vi "HandleComands.vi"(0 "Stand in":refnum<class "Stand.lvclass">, 11 "error in (no error)":errorcluster) -> (4 "Stand out":refnum<class "Stand.lvclass">, 6 "String":string, 13 "dt handle cmd":u32, 15 "error out":errorcluster)   [LabVIEW 2019, in "Stand.lvclass"]
uses:
  Stand.lvclass
  C:/Users/ANENKOV_V1/Desktop/src/Device_class/Device.lvclass
  Device_class/Device.lvclass/Device.ctl
  Proccess_class/Proccess.lvclass/Proccess.ctl
  Modbus_class/CMD REG.ctl
  Stand.lvclass/Stand.ctl
  TypeDef/CalibrationData.ctl
  TypeDef/GUI Setting Channel.ctl
  TypeDef/GUI AI Ranges.ctl
  TypeDef/Scale Data.ctl
  SV_Puplisher_class/SV_Publisher.lvclass/SV_Publisher.ctl
  fa7aa4b9-2980-448f-9ea7-f9a96ba04b16.vi
  cf98acac-72aa-4535-b835-e10be751fc5f.vi
  bfc9a858-c3a6-4d13-83b8-6384ea99c5a7.vi
  f74d70ca-5a31-43fe-8564-a719dafc7d08.vi
  9504c8ef-5d3e-4147-8f9a-94e23ec0f1f3.vi
  02f03ceb-97e6-4151-91fa-f86219b8bb60.vi
  cdc27d4a-684e-4578-89c7-fa6de6d60a20.vi
  13e1ba5d-889d-4619-89c4-93477e31edff.vi
  9c9d60f0-6a44-4683-935b-c5188c5c961e.vi
  39aaaa99-a8d8-4d9f-8d69-d9ea65c11964.vi
  1f4e3915-6da8-46a8-831b-0301257cc98b.vi
  46a8ca8a-9e53-4c5b-b4d2-ef9efb1f3638.vi
  12eadd95-888c-421b-8b03-5d7b3a747bbb.vi
  Proccess_class/GetNames.vi
  Proccess_class/GetLogger.vi
  SV_Puplisher_class/Set SV.vi/1ae5d02c-efd0-450a-8aa4-8388e25d05bc.vi
  Device_class/Device.lvclass
  C:/Users/ANENKOV_V1/Desktop/src/Proccess_class/Proccess.lvclass
  Logger_class/WriteEvent.vi
  <vilib>/addons/_JKI.lib/Serialization/JSON/Library/Unflatten From JSON String.vi
  MessageInterface_class/MessageInterface.lvclass
  FPGA_API_class/FPGA API.lvclass
  ConfigInterface_class/ConfigInterface.lvclass
  SV_Puplisher_class/SV_Publisher.lvclass
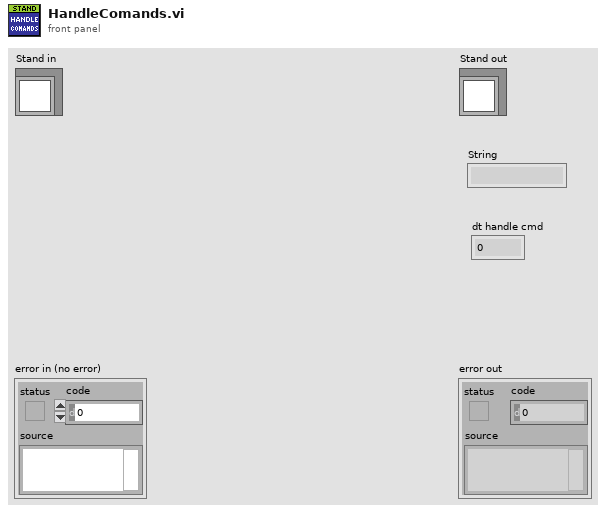
[diagram p1: front panel]
types:
  T1 = typedef "MessageInterface.lvclass/Message.ctl" = cluster{"name":string, "value":string, "receiver host":string, "receiver process":string, "source host":string, "source process":string}
  T2 = typedef "CMD REG.ctl" = cluster{"EXECUTE_SP":bool, "ALARM_PRESS_DOWN_DUT":bool, "ALARM_PRESS_DOWN_CHAMBER":bool, "ALARM_PRESS_DOWN_DUT_CHAMBER":bool, "FILING_DUT":bool, "FILING_CHAMBER":bool, "BLOCK":bool, "PUMP_STATION_OFF":bool, "Leak start":bool, "Leak stop":bool, "Drain":bool}
  T3 = typedef "CalibrationData.ctl" = cluster{"Channels":T4[], "Scales":T6[]}
  T4 = typedef "GUI Setting Channel.ctl" = cluster{"Name":string, "AI Ranges":T5, "ScaleIndex":u32}
  T5 = typedef "GUI AI Ranges.ctl" = cluster{"HI":bool, "HIHI":bool, "LO":bool, "LOLO":bool, "HIHI VAL":dbl, "HI VAL":dbl, "LO VAL":dbl, "LOLO VAL":dbl, "MAX RAW":dbl, "MIN RAW":dbl, "MAX SCALED":dbl, "MIN SCALED":dbl}
  T6 = typedef "Scale Data.ctl" = cluster{"index":i32, "Name":string, "X":dbl[], "Y":dbl[]}
  T7 = typedef "Setting Stand.ctl" = cluster{"Pressure Source":T8, "dt pressure down ms":i32, "dP pressure down MPa":dbl, "Haskel":T9, "Pump":T9, "Accuracy [%]":dbl, "Accuracy max [MPa]":dbl, "Accuracy min [MPa]":dbl, "BackPressurVoltage [V]":dbl}
  T8 = typedef "Pressure Source.ctl" = enum16{"Internal", "Modbus", "UDP"}
  T9 = typedef "Setting Pressure PI.ctl" = cluster{"A [MPa/V]":dbl, "P0 [MPa]":dbl}
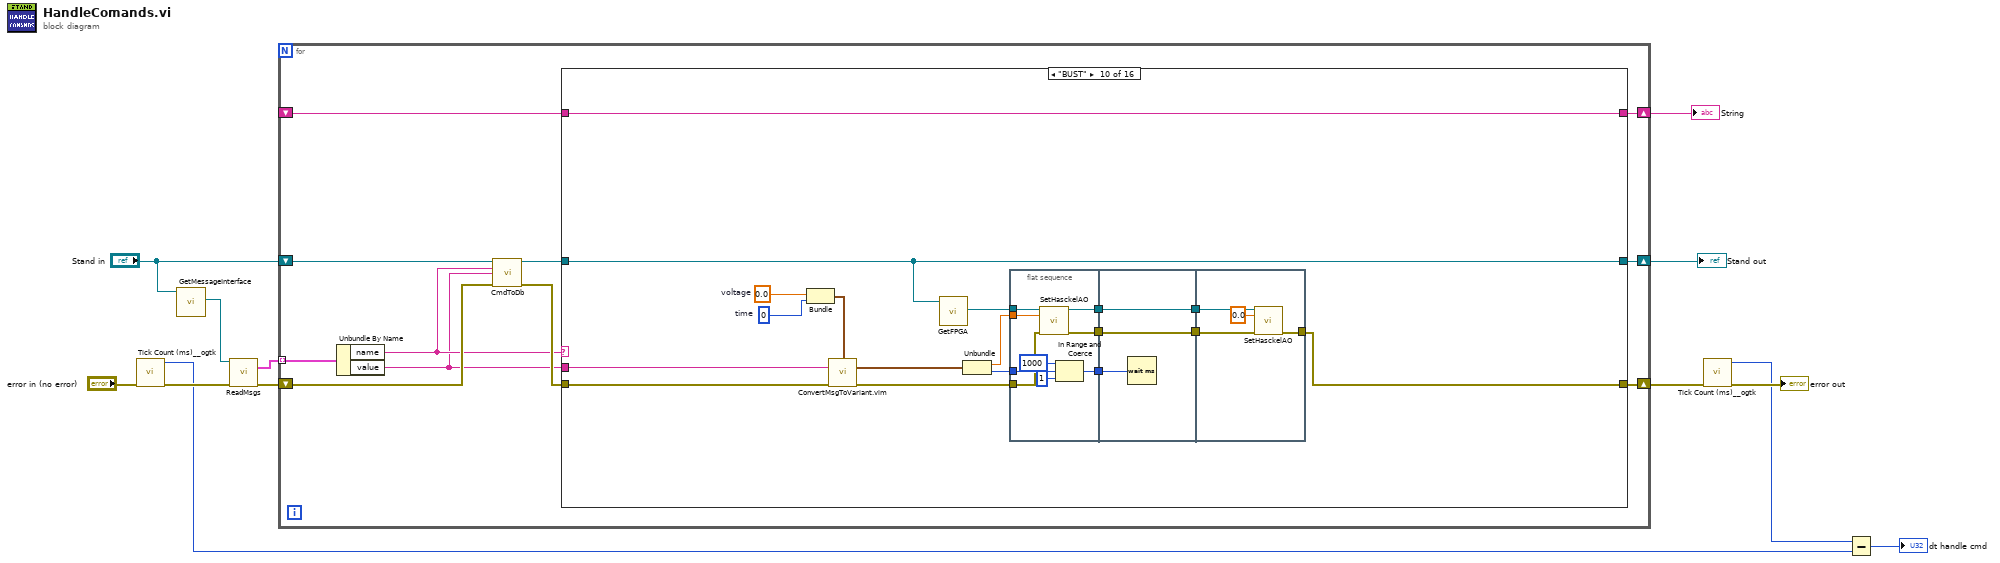
[diagram p0: block diagram]
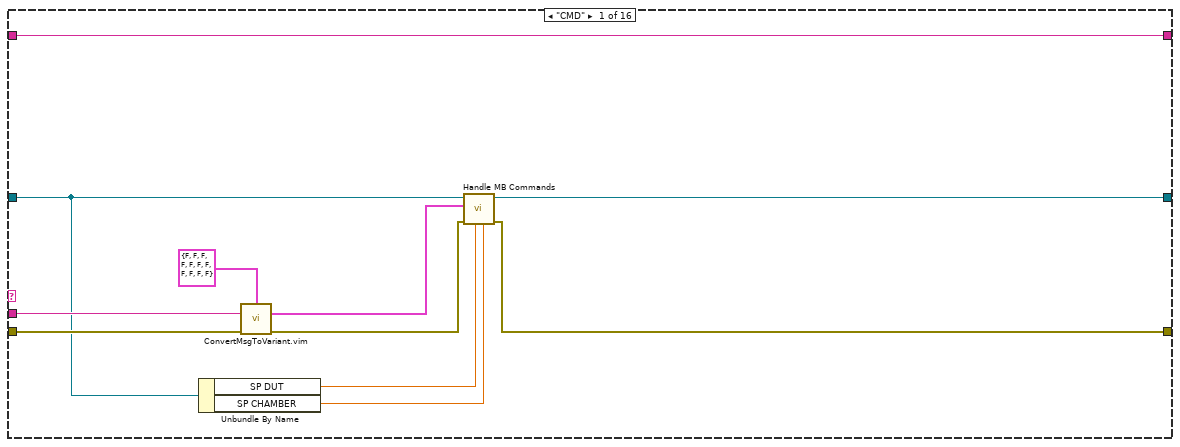
[diagram p2: hidden frame]
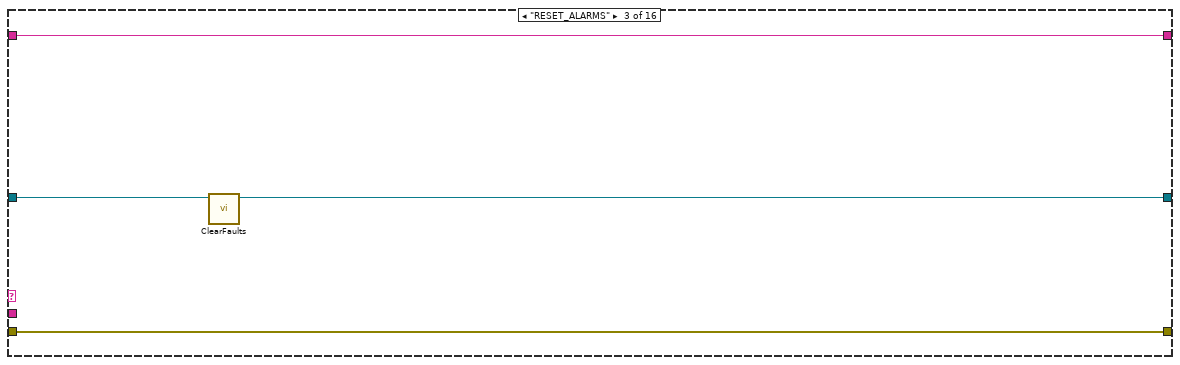
[diagram p4: hidden frame]
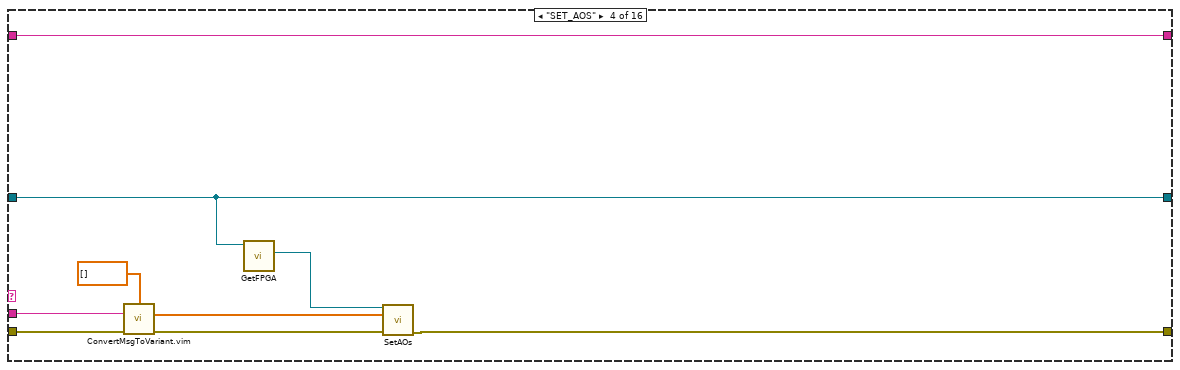
[diagram p5: hidden frame]
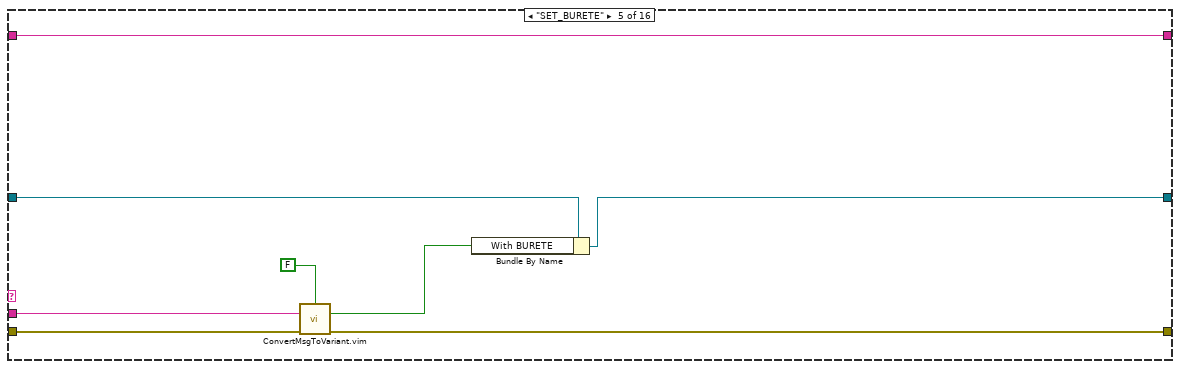
[diagram p6: hidden frame]
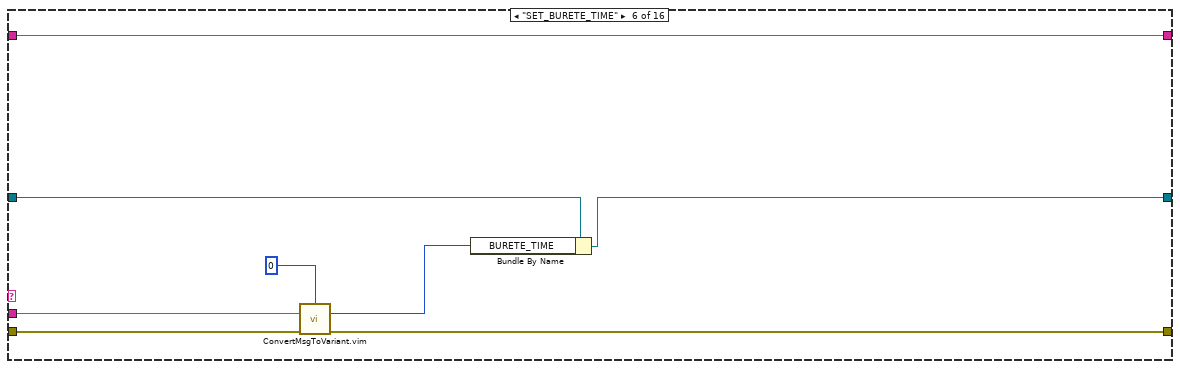
[diagram p7: hidden frame]
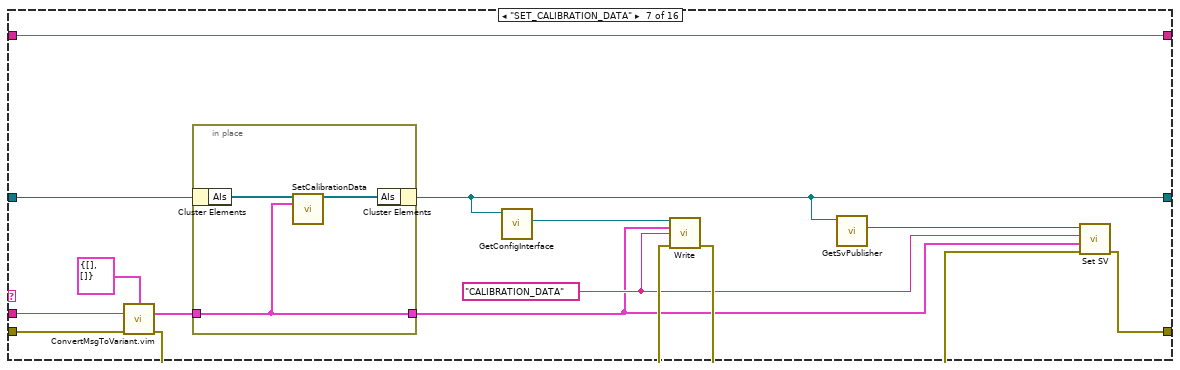
[diagram p8: hidden frame]
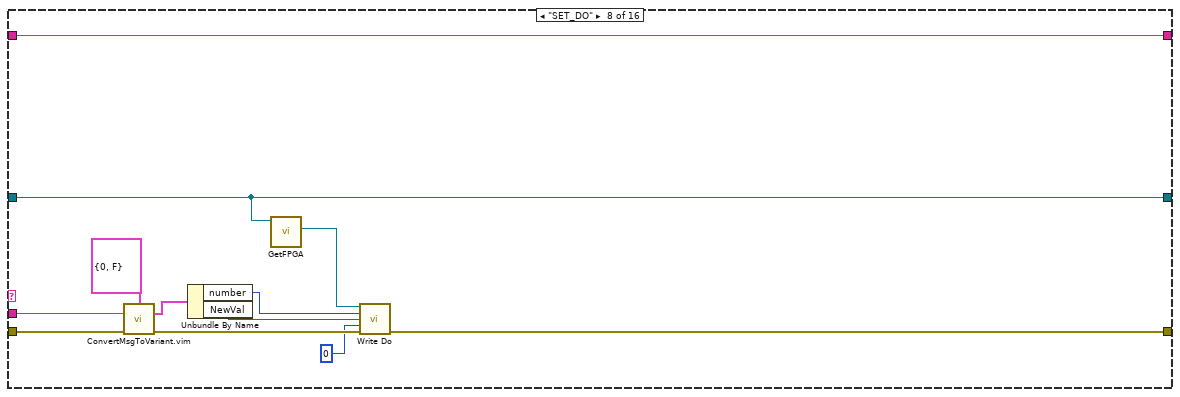
[diagram p9: hidden frame]
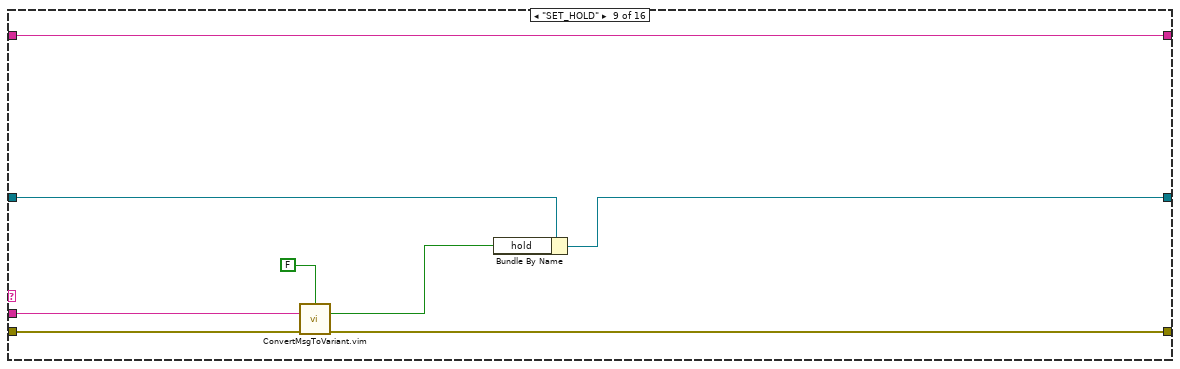
[diagram p10: hidden frame]
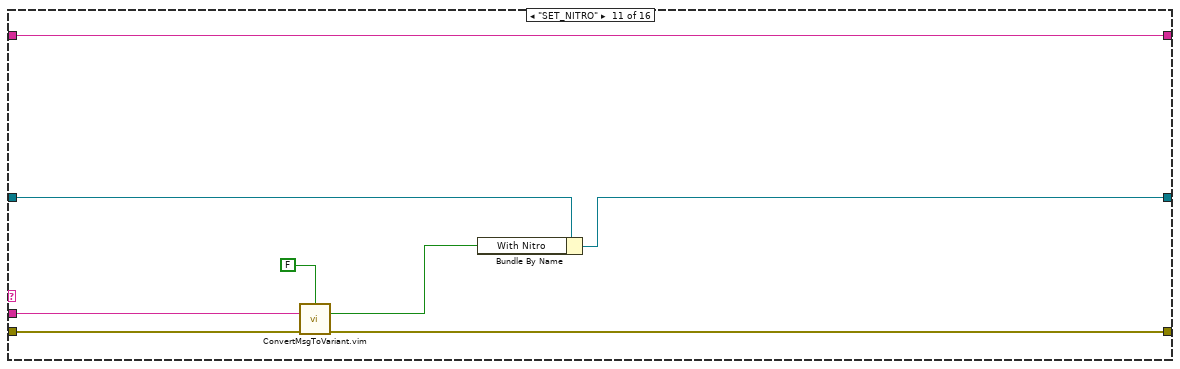
[diagram p11: hidden frame]
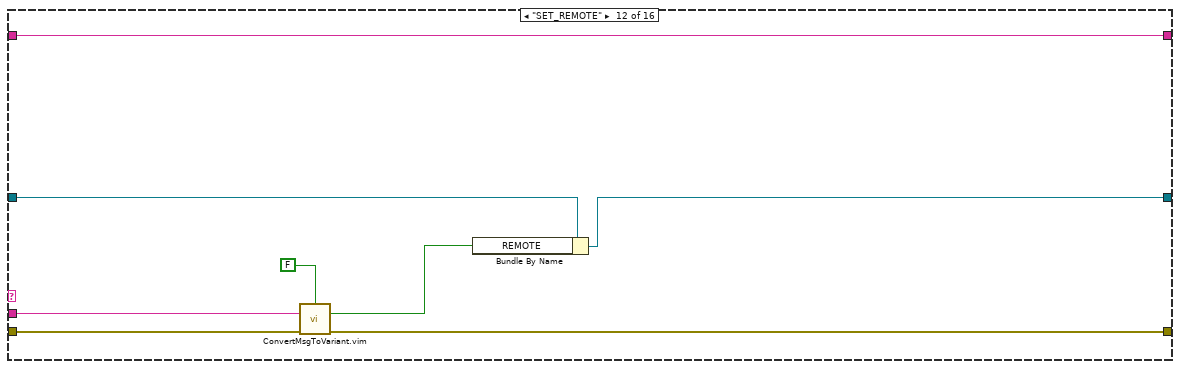
[diagram p12: hidden frame]
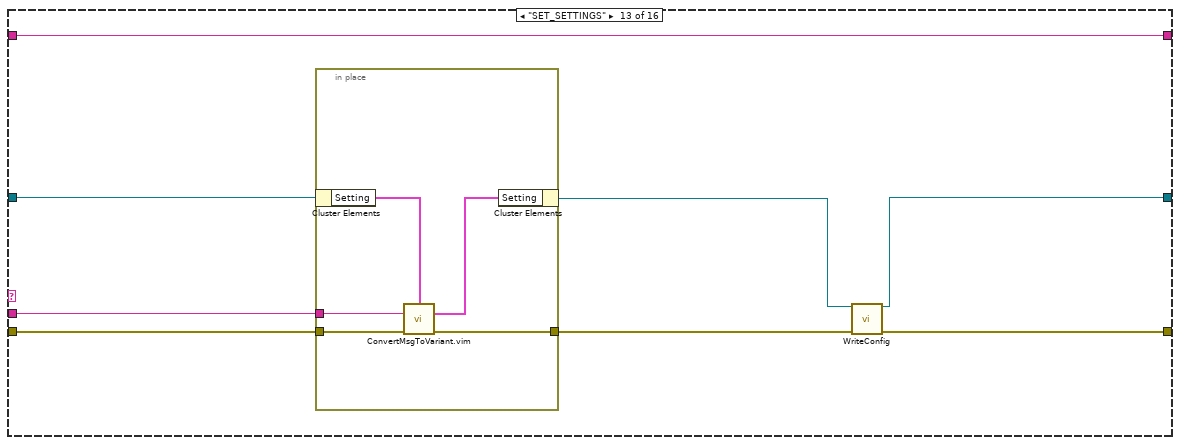
[diagram p13: hidden frame]
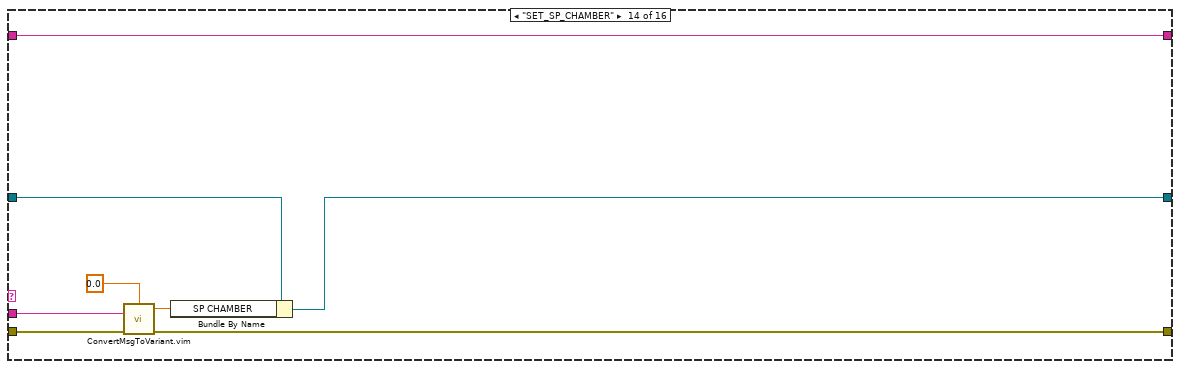
[diagram p14: hidden frame]
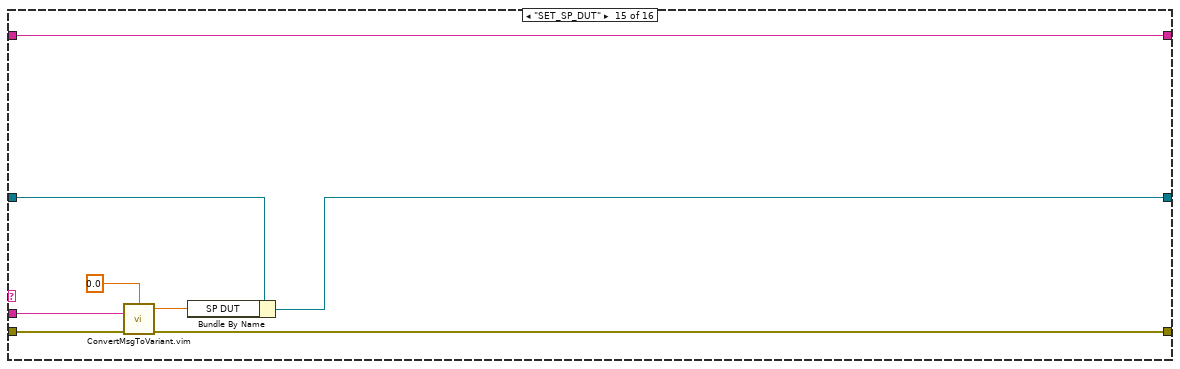
[diagram p15: hidden frame]
diagram:
  n1 = call <userlib>:"Tick Count (ms)__ogtk.vi"("error in (no error)"="error in (no error)") -> ("error out"=w6:errorcluster, "millisecond timer value"=w2:u32)  [unwired: 9 in]
  n2 = call "GetMessageInterface.vi"("Device in"="Stand in") -> ("MessageInterface"=w11:refnum<class "MessageInterface.lvclass">)  [unwired: 10 in]
  n3 = call-dynamic "ReadMsgs.vi"("reference in"=w11, "error in (no error)"=w6) -> ("msgs"=w9:T1[], "error out"=w10:errorcluster)  [unwired: 11 in, 1 out]
  n4 = for {
    shift-right: [w23] -> w4
    shift-left: w10 -> [w17]
    tunnel: w9 -> [w22] mode=indexing
    shift-right: [w24] -> w12
    shift-left: "Stand in" -> [w19]
    shift-right: [w21] -> w8
    shift-left: _ -> [w20]
    n5 = Unbundle By Name(w22) -> ("name"=w15:string, "value"=w14:string)
    n6 = call "CmdToDb.vi"("reference in"=w19, "CMD"=w15, "Value"=w14, "error in (no error)"=w17) -> ("reference out"=w18:refnum<class "Stand.lvclass">, "error out"=w16:errorcluster)  [unwired: 10 in]
    n7 = case shown="\"BUST\"" w15 {
      selector: w15 -> [_ _ _ _ _ _ _ _ _ _ _ _ _ _ _ w184]
      tunnel: [w32 w37 w41 w44 w53 w62 w74 w91 w98 w114 w140 w148 w155 w169 w177 w186] -> w24
      tunnel: w18 -> [w29 w37 w42 w44 w55 w64 w78 w91 w100 w114 w142 w150 w159 w172 w180 w186]
      tunnel: w16 -> [w33 w36 w40 w50 w58 w66 w79 w95 w103 w121 w145 w153 w161 w174 w182 w185]
      tunnel: [w25 w36 w40 w46 w54 w63 w69 w93 w99 w105 w141 w149 w157 w168 w176 w185] -> w23
      tunnel: w14 -> [w34 _ _ w51 w59 w67 w81 w96 w104 w122 w146 w154 w162 w175 w183 _]
      tunnel: [w35 w38 w39 w45 w56 w65 w68 w92 w101 w120 w143 w151 w160 w173 w181 w184] -> w21
      tunnel: w20 -> [w35 w38 w39 w45 w56 w65 w68 w92 w101 w120 w143 w151 w160 w173 w181 _]
      frame "CMD" {
        n8 = Unbundle By Name(w29) -> ("SP DUT"=w28:dbl, "SP CHAMBER"=w27:dbl)
        n9 = call "ConvertMsgToVariant.vim"("Type and Defaults"=T2 {"EXECUTE_SP"=FALSE, "ALARM_PRESS_DOWN_DUT"=FALSE, "ALARM_PRESS_DOWN_CHAMBER"=FALSE, "ALARM_PRESS_DOWN_DUT_CHAMBER"=FALSE, "FILING_DUT"=FALSE, "FILING_CHAMBER"=FALSE, "BLOCK"=FALSE, "PUMP_STATION_OFF"=FALSE, "Leak start"=FALSE, "Leak stop"=FALSE, "Drain"=FALSE} ("CMD REG"), "Value"=w34, "error in (no error)"=w33) -> ("data"=w30:T2, "error out"=w26:errorcluster)  [unwired: 11 in]
        n10 = call "Handle MB Commands.vi"("SP_CHAMBER"=w27, "SP_DUT"=w28, "error in (no error)"=w26, "CMD REG"=w30, "Stand in"=w29) -> ("error out"=w25:errorcluster, "Stand out"=w32:refnum<class "Stand.lvclass">)  [unwired: 5 in]
      }
      frame "INIT" {
      }
      frame "RESET_ALARMS" {
        n11 = call-dynamic "ClearFaults.vi"("reference in"=w42) -> ("reference out"=w41:refnum<class "Stand.lvclass">)  [unwired: 10 in]
      }
      frame "SET_AOS" {
        n12 = call "ConvertMsgToVariant.vim"("Type and Defaults"=dbl[] [], "Value"=w51, "error in (no error)"=w50) -> ("data"=w48:dbl[], "error out"=w47:errorcluster)  [unwired: 11 in]
        n13 = call "GetFPGA.vi"("Device in"=w44) -> ("FPGA API.lvclass"=w43:refnum<class "FPGA API.lvclass">)  [unwired: 10 in]
        n14 = call-dynamic "SetAOs.vi"("FPGA API in"=w43, "ao"=w48, "error in (no error)"=w47) -> ("error out"=w46:errorcluster)  [unwired: 11 in, 1 out]
      }
      frame "SET_BURETE" {
        n15 = call "ConvertMsgToVariant.vim"("Type and Defaults"=FALSE ("Boolean"), "Value"=w59, "error in (no error)"=w58) -> ("data"=w52:bool, "error out"=w54:errorcluster)  [unwired: 11 in]
        n16 = Bundle By Name(cluster=w55, "With BURETE"=w52) -> (w53:refnum<class "Stand.lvclass">)
      }
      frame "SET_BURETE_TIME" {
        n17 = call "ConvertMsgToVariant.vim"("Type and Defaults"=u16 0, "Value"=w67, "error in (no error)"=w66) -> ("data"=w61:u16, "error out"=w63:errorcluster)  [unwired: 11 in]
        n18 = Bundle By Name(cluster=w64, "BURETE_TIME"=w61) -> (w62:refnum<class "Stand.lvclass">)
      }
      frame "SET_CALIBRATION_DATA" {
        w71 = "CALIBRATION_DATA" ("Name")
        n19 = call "ConvertMsgToVariant.vim"("Type and Defaults"=T3 {"Channels"=[], "Scales"=[]} ("CalibrationData"), "Value"=w81, "error in (no error)"=w79) -> ("data"=w77:T3, "error out"=w75:errorcluster)  [unwired: 11 in]
        n20 = in-place {
          in-place-border: w77 -> [w82]
          in-place-border: [w82] -> w70
          n21 = in-place-cluster #1(w78) -> ("AIs"=w83:refnum<class "AI.lvclass">[])
          n22 = call "SetCalibrationData.vi"("AIs in"=w83, "data"=w82) -> ("AIs out"=w84:refnum<class "AI.lvclass">[])  [unwired: 13 in]
          n23 = in-place-cluster #1("AIs"=w84) -> (w74:refnum<class "Stand.lvclass">)
        }
        n24 = call "GetConfigInterface.vi"("Device in"=w74) -> ("ConfigInterface"=w76:refnum<class "ConfigInterface.lvclass">)  [unwired: 10 in]
        n25 = call-dynamic "Write.vi"("reference in"=w76, "Data"=w70, "Name"=w71, "error in (no error)"=w75) -> ("error out"=w73:errorcluster)  [unwired: 8 in, 3 out]
        n26 = call "GetSvPublisher.vi"("Device in"=w74) -> ("SV_Publisher.lvclass"=w72:refnum<class "SV_Publisher.lvclass">)  [unwired: 10 in]
        n27 = call "Set SV.vi"("error in (no error)"=w73, "SV Value"=w70, "SV Name"=w71, "SV_Publisher in"=w72) -> ("error out"=w69:errorcluster)  [unwired: 6 in, 1 out]
      }
      frame "SET_DO" {
        n28 = call "ConvertMsgToVariant.vim"("Type and Defaults"=cluster{"number":i32, "NewVal":bool} {"number"=0, "NewVal"=FALSE} ("output cluster"), "Value"=w96, "error in (no error)"=w95) -> ("data"=w87:cluster{"number":i32, "NewVal":bool}, "error out"=w94:errorcluster)  [unwired: 11 in]
        n29 = Unbundle By Name(w87) -> ("number"=w86:i32, "NewVal"=w85:bool)
        n30 = call "GetFPGA.vi"("Device in"=w91) -> ("FPGA API.lvclass"=w90:refnum<class "FPGA API.lvclass">)  [unwired: 10 in]
        n31 = call-dynamic "Write Do.vi"("FPGA API in"=w90, "#DO"=w86, "value"=w85, "Time uSec"=u32 0, "error in (no error)"=w94) -> ("error out"=w93:errorcluster)  [unwired: 9 in, 1 out]
      }
      frame "SET_HOLD" {
        n32 = call "ConvertMsgToVariant.vim"("Type and Defaults"=FALSE ("Boolean"), "Value"=w104, "error in (no error)"=w103) -> ("data"=w97:bool, "error out"=w99:errorcluster)  [unwired: 11 in]
        n33 = Bundle By Name(cluster=w100, "hold"=w97) -> (w98:refnum<class "Stand.lvclass">)
      }
      frame "BUST" {
        w117 = 0.0  # voltage
        w116 = u32 0  # time
        n34 = Bundle("voltage"=w117, "time"=w116) -> (w115:cluster{"voltage":dbl, "time":u32})  [unwired: 1 in]
        n35 = call "ConvertMsgToVariant.vim"("Type and Defaults"=w115, "Value"=w122, "error in (no error)"=w121) -> ("data"=w119:cluster{"voltage":dbl, "time":u32}, "error out"=w110:errorcluster)  [unwired: 11 in]
        n36 = call "GetFPGA.vi"("Device in"=w114) -> ("FPGA API.lvclass"=w118:refnum<class "FPGA API.lvclass">)  [unwired: 10 in]
        n37 = Unbundle(w119) -> ("voltage"=w113:dbl, "time"=w111:u32)
        n38 = flat-sequence {
          tunnel: w118 -> [w131]
          tunnel: w113 -> [w130]
          tunnel: [w125] -> w112
          tunnel: w111 -> [w129]
          tunnel: w110 -> [w128]
          tunnel: [w127] -> w108
          tunnel: [w126] -> w106
          tunnel: w112 -> [w134]
          tunnel: [w133] -> w109
          tunnel: w108 -> [w133]
          tunnel: [w132] -> w107
          tunnel: w106 -> [w132]
          tunnel: w109 -> [w138]
          tunnel: w107 -> [w137]
          tunnel: [w135] -> w105
          frame #0 {
            n39 = call-dynamic "SetHasckelAO.vi"("FPGA API in"=w131, "Haskel in"=w130, "error in (no error)"=w128) -> ("FPGA API out"=w127:refnum<class "FPGA API.lvclass">, "error out"=w126:errorcluster)  [unwired: 11 in]
            n40 = In Range and Coerce(upper limit=u32 1000, x=w129, lower limit=u32 1) -> (coerced(x)=w125:u32)  [unwired: 1 out]
          }
          frame #1 {
            n41 = Wait (ms)(milliseconds to wait=w134) -> ()  [unwired: 1 out]
          }
          frame #2 {
            n42 = call-dynamic "SetHasckelAO.vi"("FPGA API in"=w138, "Haskel in"=0.0, "error in (no error)"=w137) -> ("error out"=w135:errorcluster)  [unwired: 11 in, 1 out]
          }
        }
      }
      frame "SET_NITRO" {
        n43 = call "ConvertMsgToVariant.vim"("Type and Defaults"=FALSE ("Boolean"), "Value"=w146, "error in (no error)"=w145) -> ("data"=w139:bool, "error out"=w141:errorcluster)  [unwired: 11 in]
        n44 = Bundle By Name(cluster=w142, "With Nitro"=w139) -> (w140:refnum<class "Stand.lvclass">)
      }
      frame "SET_REMOTE" {
        n45 = call "ConvertMsgToVariant.vim"("Type and Defaults"=FALSE ("Boolean"), "Value"=w154, "error in (no error)"=w153) -> ("data"=w147:bool, "error out"=w149:errorcluster)  [unwired: 11 in]
        n46 = Bundle By Name(cluster=w150, "REMOTE"=w147) -> (w148:refnum<class "Stand.lvclass">)
      }
      frame "SET_SETTINGS" {
        n47 = in-place {
          in-place-border: w162 -> [w167]
          in-place-border: w161 -> [w166]
          in-place-border: [w165] -> w158
          n48 = in-place-cluster #2(w159) -> ("Setting"=w164:T7)
          n49 = call "ConvertMsgToVariant.vim"("Type and Defaults"=w164, "Value"=w167, "error in (no error)"=w166) -> ("data"=w163:T7, "error out"=w165:errorcluster)  [unwired: 11 in]
          n50 = in-place-cluster #2("Setting"=w163) -> (w156:refnum<class "Stand.lvclass">)
        }
        n51 = call-dynamic "WriteConfig.vi"("reference in"=w156, "error in (no error)"=w158) -> ("reference out"=w155:refnum<class "Stand.lvclass">, "error out"=w157:errorcluster)  [unwired: 12 in]
      }
      frame "SET_SP_CHAMBER" {
        n52 = call "ConvertMsgToVariant.vim"("Type and Defaults"=0.0, "Value"=w175, "error in (no error)"=w174) -> ("data"=w170:dbl, "error out"=w168:errorcluster)  [unwired: 11 in]
        n53 = Bundle By Name(cluster=w172, "SP CHAMBER"=w170) -> (w169:refnum<class "Stand.lvclass">)
      }
      frame "SET_SP_DUT" {
        n54 = call "ConvertMsgToVariant.vim"("Type and Defaults"=0.0, "Value"=w183, "error in (no error)"=w182) -> ("data"=w178:dbl, "error out"=w176:errorcluster)  [unwired: 11 in]
        n55 = Bundle By Name(cluster=w180, "SP DUT"=w178) -> (w177:refnum<class "Stand.lvclass">)
      }
      frame Default {
      }
    }
  }
  "Stand out" <- w12
  "String" <- w8
  n56 = call <userlib>:"Tick Count (ms)__ogtk.vi"("error in (no error)"=w4) -> ("error out"=→"error out":errorcluster, "millisecond timer value"=w3:u32)  [unwired: 9 in]
  n57 = Subtract(x=w3, y=w2) -> (x-y=→"dt handle cmd":u32)
